vi "Settings.vi"(8 "error in (no error)":errorcluster, 11 "CAD Dispense2 in":refnum<class "CAD Dispense2.lvclass">) -> (0 "error out":errorcluster, 3 "CAD Dispense2 out":refnum<class "CAD Dispense2.lvclass">)   [LabVIEW 2016, in "CAD Dispense2.lvclass"]
uses:
  CAD Dispense2.lvclass
panel:
  in  "Time?":bool
  in  "Pattern":u16(ring)=4 items=["6inchSKIROC", "Circle 5", "Circle 6", "HGCROCv1", "HGCROCV2", "Le Cercle Deux", "Le Cercle Quatre", "Le Cercle Un", "Le CercleTre", "Reasonable Glue", "Reasonable Glue 2", "Reasonable Glue 3", "Reasonable Glue 4", "Reasonable Glue 5", "Reasonable Glue 6", "SKIROCV2", "Will Practice"]
  in  "Glue Speed":i32=15
  in  "Move Speed":i32=30
  in  "Pressure (psi)":i64=30
  in  "Tip Height":dbl=-0.4 format="%#_13g"
  in  "Submit":bool=TRUE
  # "CAD Dispense"
  # "Tip Height:\nAcrylic : -0.5\nSensor : -0.4"
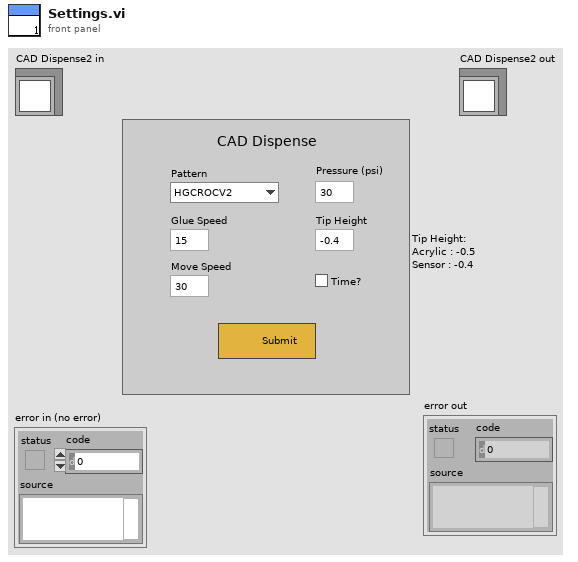
[diagram p1: front panel]
types:
  T1 = typedef "File Paths.ctl" = cluster{"Glue Pattern Folder":path, "Carrier Tray Folder":path, "Pick Up Tool Fixture Folder":path, "Components Folder":path, "Bellows Tool Offset.txt":path, "Pick Up Tool Offset.txt":path, "Dispense Tip Offset.txt":path, "Log Files":path}
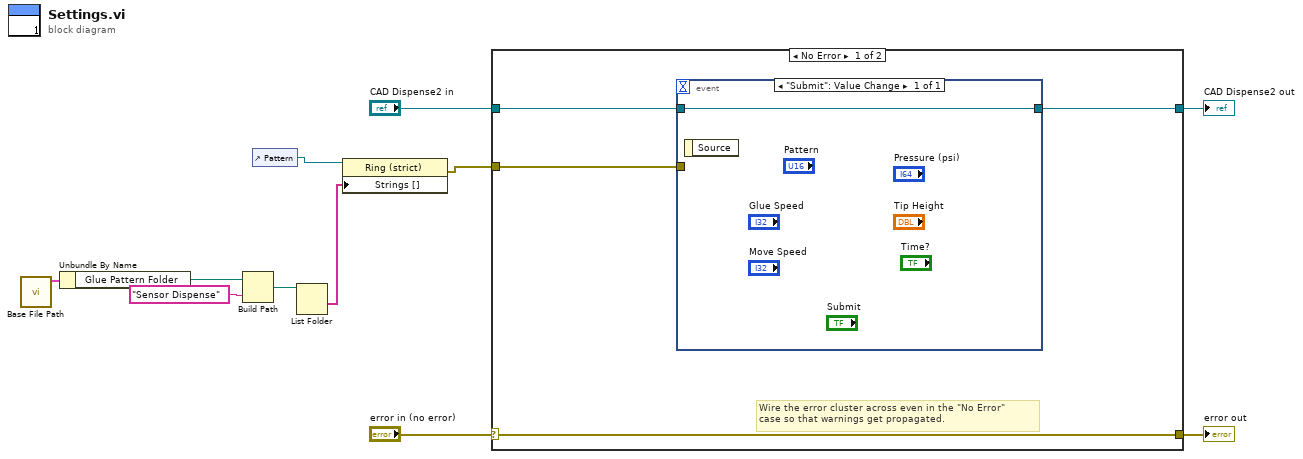
[diagram p0: block diagram]
diagram:
  n1 = call "Base File Path.vi"() -> ("Paths Out"=w7:T1)  [unwired: 11 in]
  n2 = Unbundle By Name(w7) -> ("Glue Pattern Folder"=w6:path)
  n3 = Build Path(base path=w6, name or relative path="Sensor Dispense") -> (appended path=w4:path)
  n4 = control-ref of="Pattern"() -> (w3:refnum<vi>)
  n5 = List Folder(path=w4) -> (folder names=w1:string[])  [unwired: 3 in, 3 out]
  n6 = property class="Ring (strict)"(reference=w3, "Strings []"=w1) -> (error out=w2:errorcluster)  [unwired: 1 in, 1 out]
  n7 = case shown="No Error" "error in (no error)" {
    selector: "error in (no error)" -> [w15 w18]
    tunnel: [w15 w18] -> w10
    tunnel: [w14 w17] -> w8
    tunnel: "CAD Dispense2 in" -> [w13 w17]
    tunnel: w2 -> [w12 _]
    frame No Error {
      # "Wire the error cluster across even in the \"No Error\"\ncase so that warnings get propagated."
      n8 = event shown="[0] \"Submit\": Value Change" {
        selector: _ -> [_]
        dyn-events: _ -> [_]
        timeout: _ -> [_]
        tunnel: [w16] -> w14
        tunnel: w13 -> [w16]
        tunnel: w12 -> [_]
        event "Submit": Value Change {
          n9 = event-data() -> ()  [unwired: 1 in, 1 out]
        }
      }
    }
    frame Error {
    }
  }
  "error out" <- w10
  "CAD Dispense2 out" <- w8
